vi "GUNSC_LibDetExt.vi"(5 "detext":bool, 11 "error in (no error)":errorcluster) -> (6 "return value":i32, 15 "error out":errorcluster)   [LabVIEW 2016]
uses:
  public/c/lib/libunsc.so
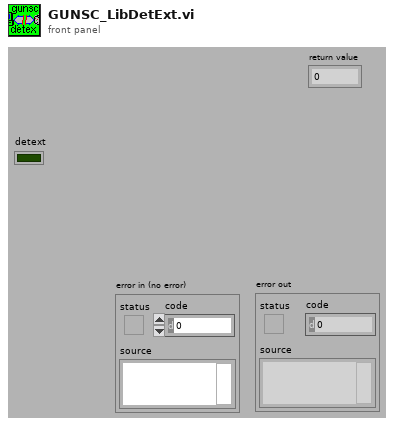
[diagram p1: front panel]
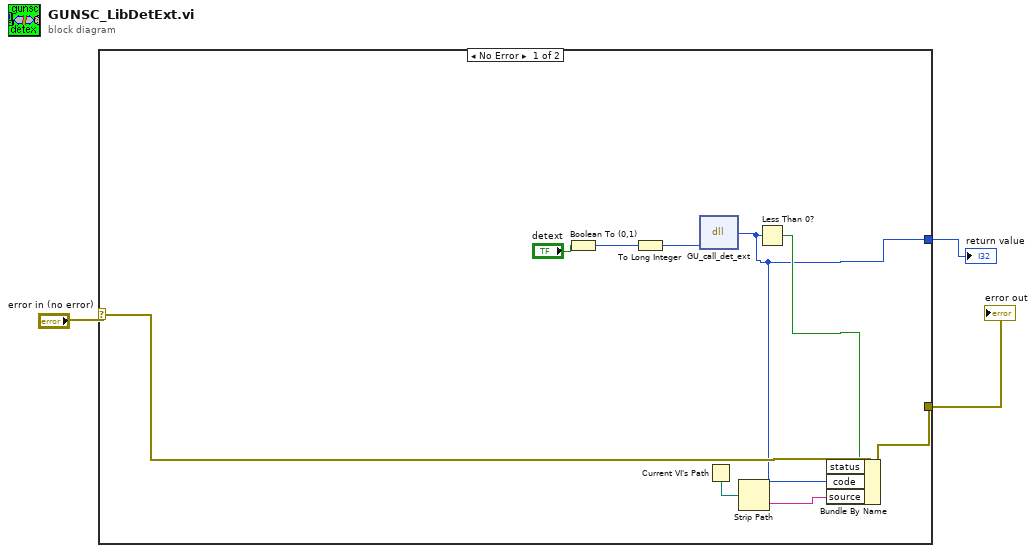
[diagram p0: block diagram]
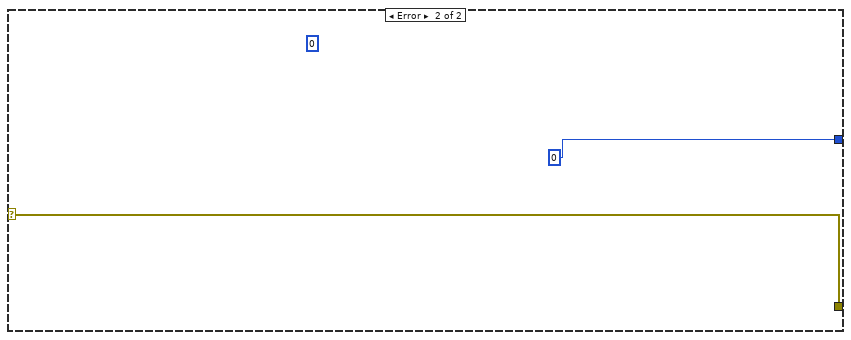
[diagram p2: hidden frame]
diagram:
  n1 = case shown="No Error" "error in (no error)" {
    selector: "error in (no error)" -> [w12 w14]
    tunnel: [w7 0] -> w3
    tunnel: [w9 w14] -> w1
    frame No Error {
      n2 = Boolean To (0,1)(Boolean="detext") -> (0, 1=w5:i16)
      n3 = To Long Integer(number=w5) -> (32bit integer=w4:i32)
      n4 = dll-call lib="home/simager/panview/PAN/Modules/GUNSC/public/c/lib/libunsc.so" fn="GU_call_det_ext"("flag"=w4) -> ("return type"=w7:i32)  [unwired: 4 in, 2 out]
      n5 = Current VI's Path() -> (path=w11:path)
      n6 = Strip Path(path=w11) -> (name=w10:string)  [unwired: 1 out]
      n7 = Less Than 0?(x=w7) -> (x < 0?=w8:bool)
      n8 = Bundle By Name(cluster=w12, "status"=w8, "code"=w7, "source"=w10) -> (w9:errorcluster)
    }
    frame Error {
      (unwired) 0
    }
  }
  "return value" <- w3
  "error out" <- w1
